vi "Actor Core.vi"(8 "error in":errorcluster, 11 "Business Logic in":refnum<class "Business Logic.lvclass">) -> (0 "error out":errorcluster, 3 "Actor out":refnum<class "Actor.lvclass">)   [LabVIEW 2020, in "Business Logic.lvlib" / "Business Logic.lvclass"]
doc: "(<B>Filename</B>: Actor Framework.lvlib:Actor.lvclass:Actor Core.vi)\n\nReceives messages to the actor, reacts to them, and initiates any error handling that may shut the actor down.\n\nDescendant classes may override this VI to append parallel tasks for the actor to complete while it handles messages. Overrides use the Call Parent Class Method node."
uses:
  Business Logic.lvclass
  C:/Program Files (x86)/National Instruments/LabVIEW 2020/vi.lib/ActorFramework/Actor/Actor.lvclass
  <vilib>/ActorFramework/Actor/Actor.lvclass
  User Interface/User Interface.lvclass
  Linear Encoder/Linear Encoder.lvclass
  Business Logic.lvclass/Business Logic.ctl
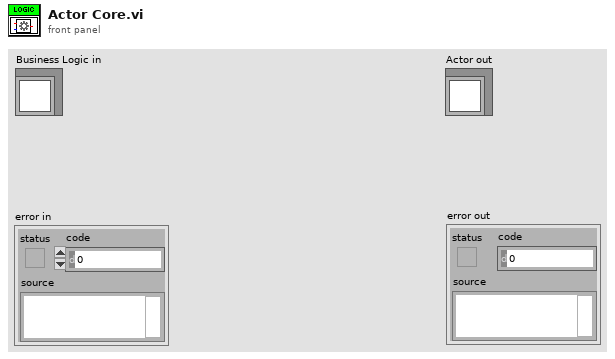
[diagram p1: front panel]
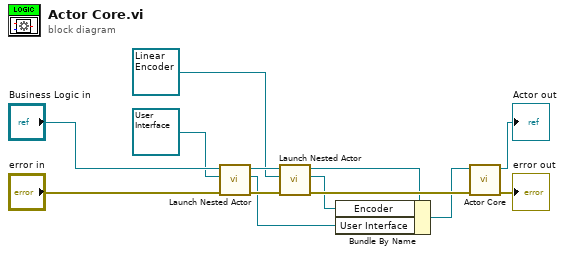
[diagram p0: block diagram]
diagram:
  n1 = call <vilib>:"Launch Nested Actor.vi"("error in (no error)"="error in", "Nested Actor"=refnum<class "User Interface.lvclass"> refnum ("User Interface.lvlib:User Interface.lvclass"), "Caller Actor in"="Business Logic in") -> ("error out"=w10:errorcluster, "Nested Actor's Enqueuer"=w1:refnum<class "Message Enqueuer.lvclass">, "Caller Actor out"=w7:refnum<class "Business Logic.lvclass">)  [unwired: 6 in]
  n2 = call <vilib>:"Launch Nested Actor.vi"("error in (no error)"=w10, "Nested Actor"=refnum<class "Linear Encoder.lvclass"> refnum ("Linear Encoder.lvlib:Linear Encoder.lvclass"), "Caller Actor in"=w7) -> ("error out"=w8:errorcluster, "Nested Actor's Enqueuer"=w2:refnum<class "Message Enqueuer.lvclass">, "Caller Actor out"=w6:refnum<class "Business Logic.lvclass">)  [unwired: 6 in]
  n3 = Bundle By Name(cluster=w6, "Encoder"=w2, "User Interface"=w1) -> (w3:refnum<class "Business Logic.lvclass">)
  n4 = call-parent "Actor Core.vi"("error in"=w8, "Actor in"=w3) -> ("error out"=→"error out":errorcluster, "Actor out"=→"Actor out":refnum<class "Actor.lvclass">)  [unwired: 8 in]
